vi "Debug.vi"() -> ()   [LabVIEW 2023]
panel:
  in  "stop":bool
  in  "Abort?":bool
  in  "Visible":bool
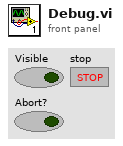
[diagram p1: front panel]
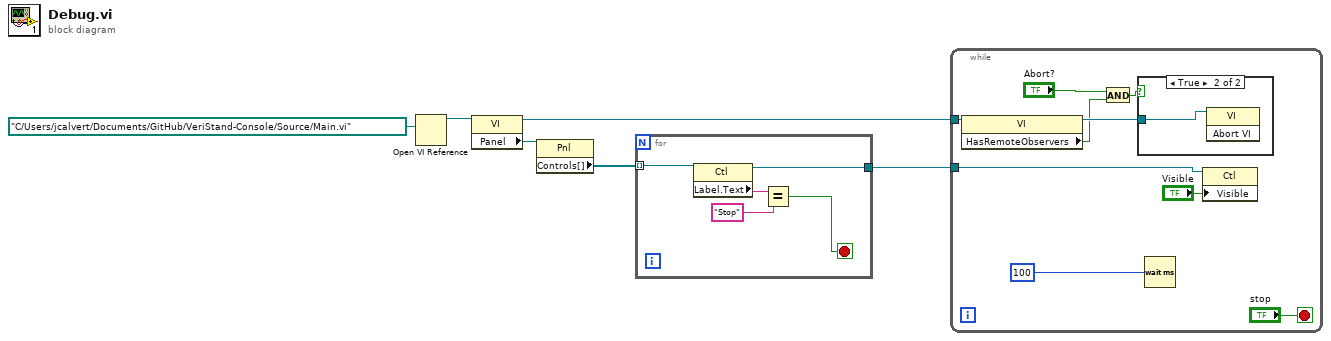
[diagram p0: block diagram]
diagram:
  n1 = Open VI Reference(vi path=path "C:/Users/jcalvert/Documents/GitHub/VeriStand-Console/Source/Main.vi") -> (vi reference=w5:refnum<vi>)  [unwired: 5 in, 1 out]
  n2 = property class="VI"(reference=w5) -> (reference out=w1:refnum<vi>, "Panel"=w4:refnum<vi>)  [unwired: 1 in, 1 out]
  n3 = property class="Pnl"(reference=w4) -> ("Controls[]"=w3:refnum<vi>[])  [unwired: 1 in, 2 out]
  n4 = for {
    tunnel: w3 -> [w11] mode=indexing
    tunnel: [w7] -> w2
    stop <- w8 stop-if-true
    n5 = property class="Ctl"(reference=w11) -> (reference out=w7:refnum<vi>, "Label.Text"=w10:string)  [unwired: 1 in, 1 out]
    n6 = Equal?(x=w10, y="Stop") -> (x = y?=w8:bool)
  }
  n7 = while {
    tunnel: w2 -> [w20]
    tunnel: w1 -> [w18]
    stop <- "stop" stop-if-true
    n8 = property class="VI"(reference=w18) -> (reference out=w14:refnum<vi>, "HasRemoteObservers"=w12:bool)  [unwired: 1 in, 1 out]
    n9 = And(x="Abort?", y=w12) -> (x .and. y?=w13:bool)
    n10 = case shown="True" w13 {
      tunnel: w14 -> [_ w21]
      frame False {
      }
      frame True {
        n11 = invoke class="VI" method="Abort VI"(reference=w21) -> ()  [unwired: 2 in, 3 out]
      }
    }
    n12 = Wait (ms)(milliseconds to wait=u32 100) -> ()  [unwired: 1 out]
    n13 = property class="Ctl"(reference=w20, "Visible"="Visible") -> ()  [unwired: 1 in, 2 out]
  }
